vi "Front Panel.vi"(11 "GUI In":refnum<class "Humidity Profile UI.lvclass">) -> ()   [LabVIEW 2015, in "Humidity Profile UI.lvclass"]
uses:
  Humidity Profile UI.lvclass
  Seq.ctl
  Humidity Profile/Change Temperature/Change Temperature.lvclass
  Reusable/GUI/GUI.lvclass/GUI.ctl
  Reusable/Observer/Observer.lvclass/Observer.ctl
  Reusable/Sequence/SEQ/SEQ.lvclass
  Reusable/Sequence/STEPS/STEP.lvclass
  Humidity Profile/Change PAS Flow/Change PAS Flow.lvclass
  Reusable/Sequence/STEPS/LEAVES/Double/Switch DBL.lvclass/Switch DBL.ctl
  Humidity Profile/Change QmRH/Change QmRH.lvclass
  Calibration/Change Filter State/Change Filter Position.lvclass
  Humidity Profile/Change Flow/Change Flow.lvclass
  Calibration/Wait/Wait.lvclass
  Calibration/Wait/Wait.lvclass/Wait.ctl
  Controls/MFC Address.ctl
  CRDS/Data/cCRDS Data.lvclass
  Reusable/Sequence/STEPS/LEAVES/Double/Write val.vi
  Calibration/Wait/Write Wait Time.vi
  Reusable/GUI/Accessors/Read RegEvent.vi
  Reusable/Observer/Read Data Queue.vi
  CRDS/Data/Read vData.vi
  CRDS/Data/Read Humidifier T.vi
  Reusable/Data/Data.lvclass
panel:
  in  "cSequence":bool
  in  "lSequence":bool
  in  "saveSeq":bool
  out "Alicat Data":T1
  out "T":sgl
  in  "run":bool
  in  "T":sgl caption="T (degC)"
  in  "Q":sgl caption="Qclap (lpm)"
  out "seqMsg":string[](array[string]) caption="Messages"
  in  "Steps":string[](tree)
  in  "Sequence":string(tree)
  # "This user interface is used to handle the profiling of humidities.  The system handles three different humidified channels.  The temperature handled on this page is the temperature associated with the medium RH channel.  The flow controls the dilution flow to the mixing tank between the high humidity channel and the channel that the thermal denuded channel.  This flow is directly connected to the high humidity flow control on the CRD page."
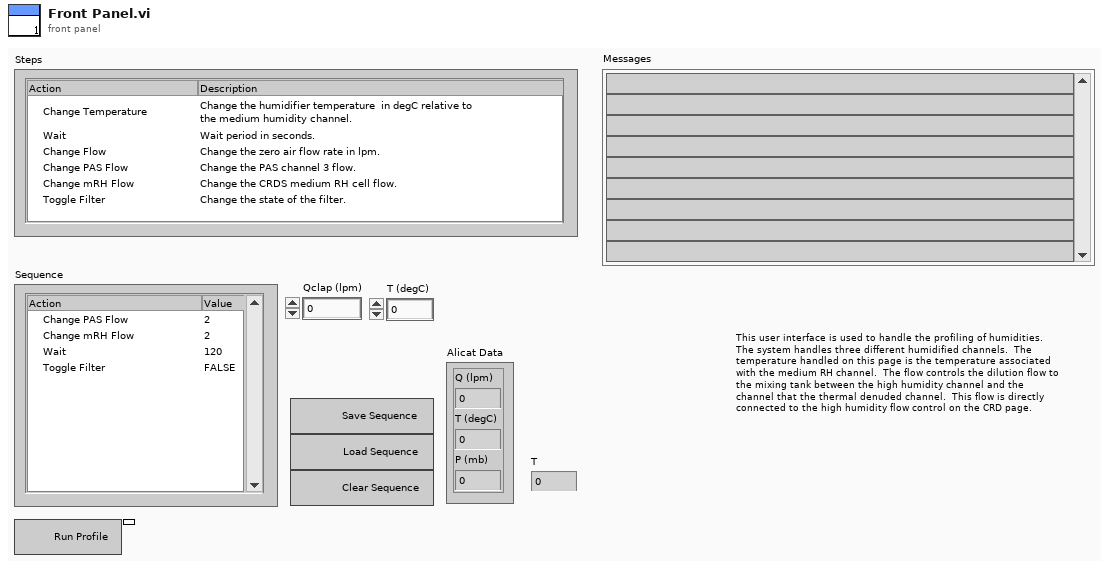
[diagram p1: front panel]
types:
  T1 = cluster{"Q (lpm)":dbl, "T (degC)":dbl, "P (mb)":dbl}
  T2 = typedef "Seq.ctl" = enum16{"Load Sequence", "Run Sequence", "Stop Sequence", "Do Nothing"}
  T3 = cluster{"Numeric":sgl, "Numeric":sgl, "Numeric":sgl}
  T4 = typedef "eventvkey.ctl" = enum16{"ASCII", "Enter", "Return", "Shift", "Ctrl", "Alt", "Cmd", "Opt", "Caps", "NumLock", "Clear", "Break", "Up", "Down", "Left", "Right", "Insert", "Delete", "Home", "End", "PageUp", "PageDown", "Escape", "Help", "Pause", "ScrollLock", "F1", "F2", "F3", "F4", "F5", "F6", "F7", "F8", "F9", "F10", "F11", "F12", "F13", "F14", "F15", "F16", "F17", "F18", "F19", "F20", "F21", "F22", "F23", "F24", "Play", "VolumeUp", "VolumeDown", "Mute", "Two Byte Char"}
  T5 = enum16{"Load Sequence", "Run Sequence", "Stop Sequence"}
  T6 = typedef "MFC Address.ctl" = enum16{"CRDS Purge", "CRDS Thermodenuded", "CRDS Dry", "CRDS Med RH", "CRDS High RH", "PAS Ch 1", "PAS Ch 2", "PAS Ch3", "PAS Ch 4", "PAS Ch 5", "CLAP", "O3", "Pinlet"}
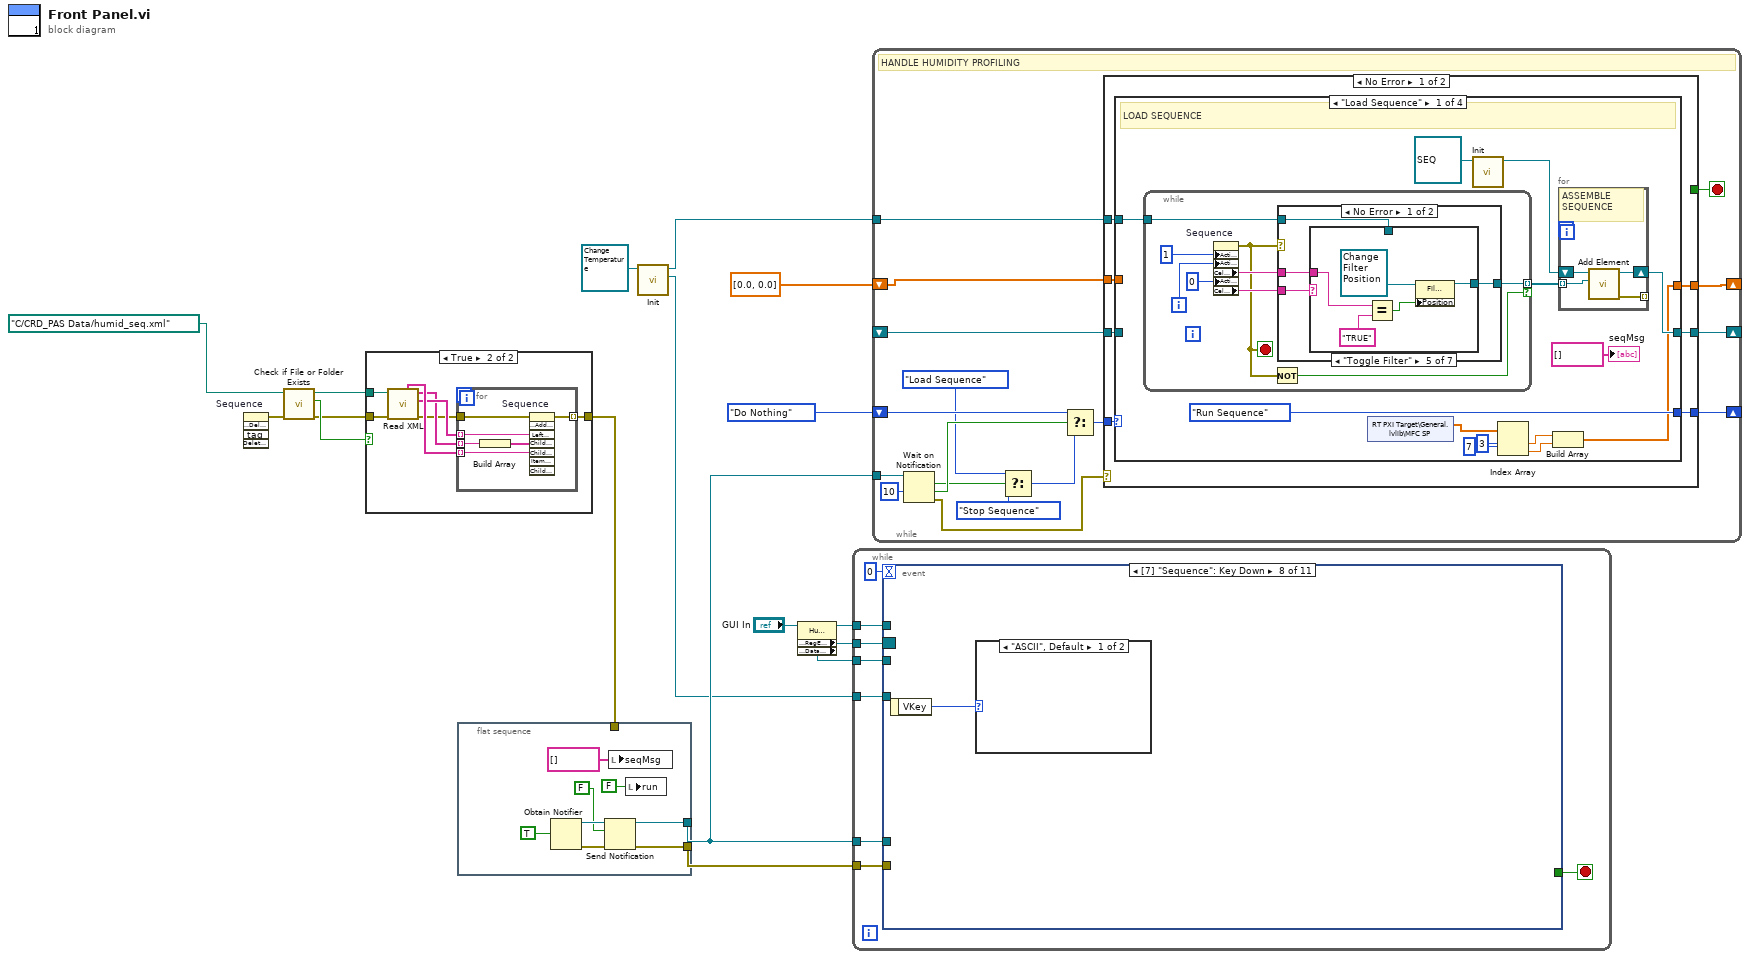
[diagram p0: block diagram]
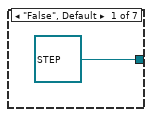
[diagram p3: hidden frame]
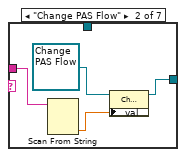
[diagram p4: hidden frame]
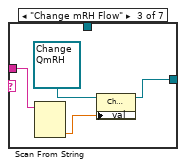
[diagram p5: hidden frame]
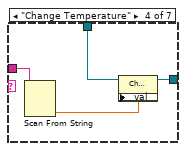
[diagram p6: hidden frame]
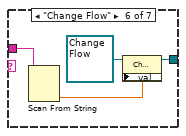
[diagram p7: hidden frame]
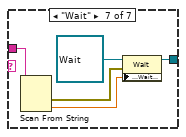
[diagram p8: hidden frame]
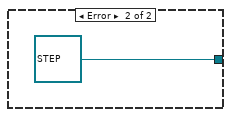
[diagram p9: hidden frame]
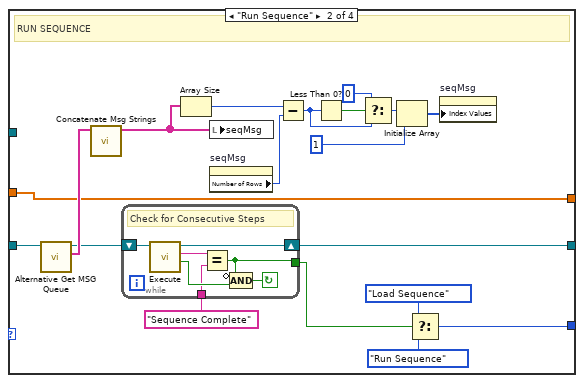
[diagram p10: hidden frame]
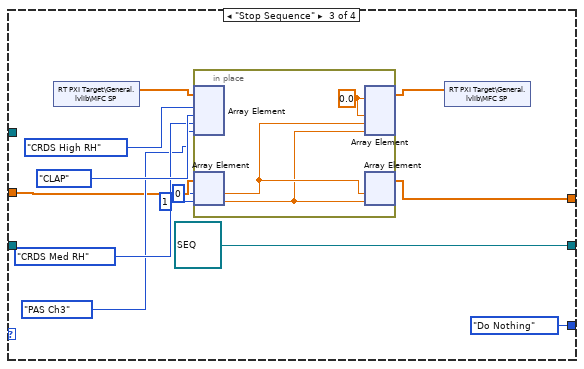
[diagram p11: hidden frame]
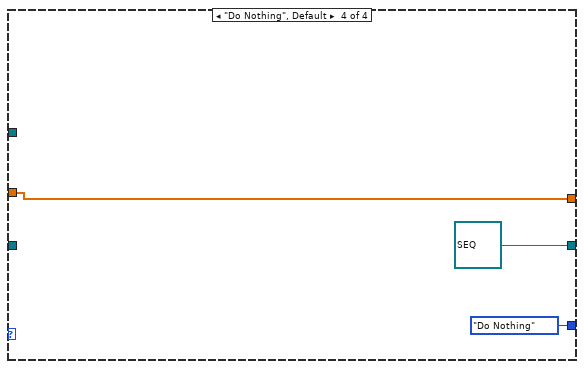
[diagram p12: hidden frame]
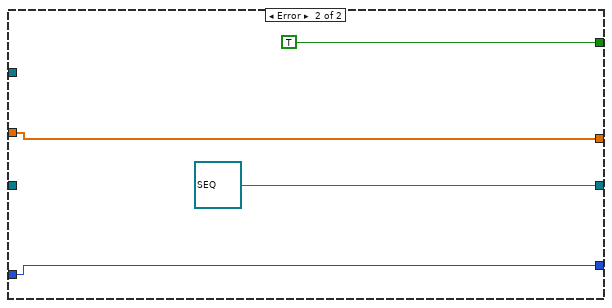
[diagram p13: hidden frame]
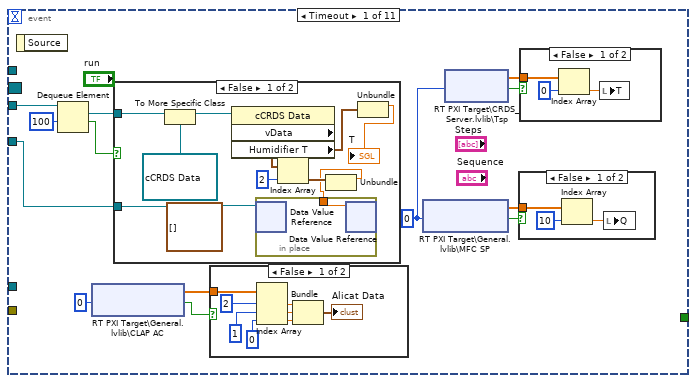
[diagram p14: hidden frame]
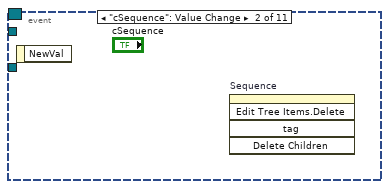
[diagram p19: hidden frame]
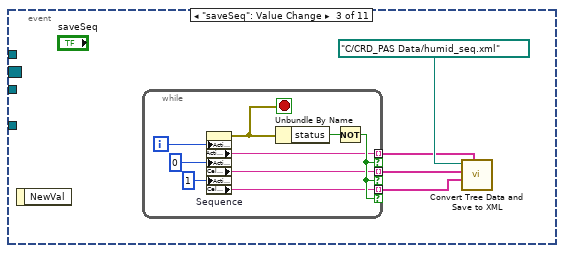
[diagram p20: hidden frame]
diagram:
  n1 = invoke on="Sequence" class="Tree (strict)" method="Edit Tree Items.Delete"() -> (error out=w9:errorcluster)  [unwired: 5 in, 4 out]
  n2 = call <vilib>:"Check if File or Folder Exists.vi"("error in (no error)"=w9, "path"=path "C:/CRD_PAS Data/humid_seq.xml" ("file")) -> ("error out"=w8:errorcluster, "file or folder exists?"=w10:bool, "dup path"=w7:path)  [unwired: 7 in]
  n3 = case shown="True" w10 {
    tunnel: w8 -> [_ w20]
    tunnel: w7 -> [_ w22]
    tunnel: [_ w18] -> w5
    frame False {
    }
    frame True {
      n4 = call "Read XML.vi"("error in"=w20, "path"=w22) -> ("error out"=w19:errorcluster, "Steps"=w23:string[], "Values"=w21:string[], "tags"=w24:string[])  [unwired: 5 in, 1 out]
      n5 = for {
        tunnel: w24 -> [w30] mode=indexing
        tunnel: w23 -> [w29] mode=indexing
        tunnel: w21 -> [w28] mode=indexing
        tunnel: w19 -> [w26]
        tunnel: [w25] -> w18 mode=indexing
        n6 = Build Array(w28) -> (w27:string[])
        n7 = invoke on="Sequence" class="Tree (strict)" method="Edit Tree Items.Add Item to End"(error in=w26, "Left Cell"=w29, "Child Text"=w27, "Child Tag"=w30) -> (error out=w25:errorcluster)  [unwired: 4 in, 7 out]
      }
    }
  }
  n8 = flat-sequence {
    tunnel: [w34] -> w14
    tunnel: [w33] -> w13
    tunnel: w5 -> [_]
    frame #0 {
      n9 = Obtain Notifier(notification data type=TRUE) -> (notifier out=w37:refnum<notifier>, error out=w36:errorcluster)  [unwired: 3 in, 1 out]
      n10 = Send Notification(notification=FALSE, notifier=w37, error in (no error)=w36) -> (notifier out=w33:refnum<notifier>, error out=w34:errorcluster)
      n11 = local write "seqMsg"(string[] [] ("seqMsg")) -> ()
      n12 = local write "run"(FALSE ("run")) -> ()
    }
  }
  n13 = call "Init.vi"("Change Temperature in"=refnum<class "Change Temperature.lvclass"> refnum) -> ("T DVR"=w2:refnum<data-value>, "Change Temperature out"=w3:refnum<class "Change Temperature.lvclass">)  [unwired: 8 in, 1 out]
  n14 = property class="Humidity Profile"(reference="GUI In") -> (reference out=w11:refnum<class "Humidity Profile UI.lvclass">, "Data Access:RegEvent"=w16:refnum<event-registration>, "Data Access:Data Queue"=w15:refnum<queue>)  [unwired: 1 in, 1 out]
  n15 = while {
    tunnel: w16 -> [w46]
    tunnel: w15 -> [w44]
    tunnel: w13 -> [w43]
    tunnel: w14 -> [w42]
    tunnel: w11 -> [w40]
    tunnel: w2 -> [w39]
    stop <- w45 stop-if-true
    n16 = event shown="[7] \"Sequence\": Key Down" {
      selector: w46 -> [_ _ _ _ _ _ _ _ _ _ _]
      dyn-events: _ -> [_ _ _ _ _ _ _ _ _ _ _]
      timeout: 0 -> [_ _ _ _ _ _ _ _ _ _ _]
      tunnel: [_ _ _ _ _ _ _ _ TRUE _ _] -> w45
      tunnel: w44 -> [w59 _ _ _ _ _ _ _ _ _ _]
      tunnel: w43 -> [_ _ _ _ w119 _ _ _ w136 _ _]
      tunnel: w42 -> [_ _ _ _ w118 _ _ _ w135 _ _]
      tunnel: w40 -> [_ _ _ _ _ _ _ _ w134 _ _]
      tunnel: w39 -> [w47 _ _ _ _ _ _ _ w133 _ _]
      event Timeout {
        w52 = 0 ("ms timeout (0)")
        n17 = event-data() -> ()  [unwired: 1 in, 1 out]
        n18 = Dequeue Element(queue=w59, timeout in ms (-1)=100) -> (element=w58:refnum<data-value>, timed out?=w53:bool)  [unwired: 1 in, 2 out]
        n19 = shared-variable "RT PXI Target\\General.lvlib\\CLAP AC"(0 ("ms timeout (0)")) -> (w51:sgl[], w49:bool)  [unwired: 1 in, 1 out]
        n20 = case shown="False" w53 {
          tunnel: w58 -> [w77 _]
          tunnel: w47 -> [w74 _]
          frame False {
            (unwired) cluster{"TRH":dbl, "RH":dbl}[] [] ("vData")
            n21 = To More Specific Class(target class=refnum<data-value> refnum ("element"), reference=w77) -> (specific class reference=w75:refnum<data-value>)  [unwired: 1 in, 1 out]
            n22 = property class="cCRDS Data"(reference=w75) -> ("vData"=w73:cluster{"TRH":dbl, "RH":dbl}[], "Humidifier T"=w69:cluster{"Hum 1":sgl, "Hum 2":sgl})  [unwired: 1 in, 2 out]
            n23 = Index Array(array=w73, index=2) -> (element=w71:cluster{"TRH":dbl, "RH":dbl})
            n24 = Unbundle(w71) -> ("TRH"=w70:dbl)  [unwired: 1 out]
            n25 = in-place {
              in-place-border: w70 -> [w78]
              n26 = in-place-dvr #1(w74) -> ()  [unwired: 2 out]
              n27 = in-place-dvr #1(w78) -> ()  [unwired: 2 out]
            }
            n28 = Unbundle(w69) -> ("Hum 1"=→"T":sgl)  [unwired: 1 out]
          }
          frame True {
          }
        }
        n29 = case shown="False" w49 {
          tunnel: w51 -> [w61 _]
          frame False {
            n30 = Index Array(array=w61, index #1=2 ("index"), index #2=1 ("index"), index #3=0 ("index")) -> (element #1=w65:sgl, element #2=w66:sgl, element #3=w67:sgl)
            n31 = Bundle("Numeric"=w65, "Numeric"=w66, "Numeric"=w67) -> (→"Alicat Data":T3)  [unwired: 1 in]
          }
          frame True {
          }
        }
        n32 = shared-variable "RT PXI Target\\General.lvlib\\MFC SP"(w52) -> (w54:sgl[], w55:bool)  [unwired: 1 in, 1 out]
        n33 = shared-variable "RT PXI Target\\CRDS_Server.lvlib\\Tsp"(w52) -> (w56:sgl[], w57:bool)  [unwired: 1 in, 1 out]
        n34 = case shown="False" w55 {
          tunnel: w54 -> [w81 _]
          frame False {
            n35 = Index Array(array=w81, index=10) -> (element=w79:sgl)
            n36 = local write "Q"(w79) -> ()
          }
          frame True {
          }
        }
        n37 = case shown="False" w57 {
          tunnel: w56 -> [w84 _]
          frame False {
            n38 = Index Array(array=w84, index=0) -> (element=w82:sgl)
            n39 = local write "T"(w82) -> ()
          }
          frame True {
          }
        }
      }
      event "cSequence": Value Change {
        n40 = event-data() -> ()  [unwired: 1 in, 1 out]
        n41 = invoke on="Sequence" class="Tree (strict)" method="Edit Tree Items.Delete"() -> ()  [unwired: 5 in, 5 out]
      }
      event "saveSeq": Value Change {
        n42 = event-data() -> ()  [unwired: 1 in, 1 out]
        n43 = while {
          tunnel: [w93] -> w87 mode=indexing if=w94
          tunnel: [w90] -> w86 mode=indexing if=w94
          tunnel: [w89] -> w85 mode=indexing if=w94
          i -> [w92]
          stop <- w96 stop-if-true
          n44 = property on="Sequence" class="Tree (strict)"("Active Item Row Number"=w92, "ActiveColNum"=0 ("Active Cell:Active Column Number"), "ActiveColNum"=1 ("Active Cell:Active Column Number")) -> (error out=w96:errorcluster, "Active Item Tag"=w93:string, "Cell String"=w90:string, "Cell String"=w89:string)  [unwired: 2 in, 1 out]
          n45 = Unbundle By Name(w96) -> ("status"=w97:bool)
          n46 = Not(x=w97) -> (.not. x?=w94:bool)
        }
        n47 = call "Convert Tree Data and Save to XML.vi"("tag"=w87, "Value"=w85, "Step"=w86, "file"=path "C:/CRD_PAS Data/humid_seq.xml") -> ()  [unwired: 5 in, 3 out]
      }
      event "lSequence": Value Change {
        n48 = event-data() -> ()  [unwired: 1 in, 1 out]
        n49 = call "File Dialog"("prompt"="Open sequence file.", "pattern (all files)"="*.xml") -> ("selected path"=w101:path, "cancelled"=w99:bool, "error out"=w98:errorcluster)  [unwired: 10 in, 1 out]
        n50 = case shown="False" w99 {
          tunnel: w101 -> [w108 _]
          tunnel: [w105 _] -> _
          tunnel: w98 -> [w104 _]
          frame False {
            n51 = invoke on="Sequence" class="Tree (strict)" method="Edit Tree Items.Delete"(error in=w104) -> (error out=w103:errorcluster)  [unwired: 4 in, 4 out]
            n52 = call "Read XML.vi"("error in"=w103, "path"=w108) -> ("error out"=w106:errorcluster, "Steps"=w109:string[], "Values"=w107:string[], "tags"=w110:string[])  [unwired: 5 in, 1 out]
            n53 = for {
              tunnel: w110 -> [w116] mode=indexing
              tunnel: w109 -> [w115] mode=indexing
              tunnel: w107 -> [w114] mode=indexing
              tunnel: w106 -> [w112]
              tunnel: [w111] -> w105 mode=indexing
              n54 = Build Array(w114) -> (w113:string[])
              n55 = invoke on="Sequence" class="Tree (strict)" method="Edit Tree Items.Add Item to End"(error in=w112, "Left Cell"=w115, "Child Text"=w113, "Child Tag"=w116) -> (error out=w111:errorcluster)  [unwired: 4 in, 7 out]
            }
          }
          frame True {
          }
        }
      }
      event "run": Value Change {
        n56 = event-data() -> ("NewVal"=w117:bool)  [unwired: 1 in]
        n57 = Send Notification(notification=w117, notifier=w119, error in (no error)=w118) -> ()  [unwired: 2 out]
      }
      event "Q": Value Change {
        n58 = event-data() -> ()  [unwired: 1 in, 1 out]
        n59 = shared-variable "RT PXI Target\\General.lvlib\\MFC SP"() -> (w122:sgl[])  [unwired: 1 in, 1 out]
        n60 = in-place {
          in-place-border: "Q" -> [w124]
          n61 = in-place-array #2(w122, 10) -> ()  [unwired: 1 out]
          n62 = in-place-array #2(w124) -> (w120:sgl[])  [unwired: 1 out]
        }
        n63 = shared-variable "RT PXI Target\\General.lvlib\\MFC SP"(w120) -> ()  [unwired: 1 in, 1 out]
      }
      event "T": Value Change {
        n64 = event-data() -> ()  [unwired: 1 in, 1 out]
        n65 = shared-variable "RT PXI Target\\CRDS_Server.lvlib\\Tsp"() -> (w128:sgl[])  [unwired: 1 in, 1 out]
        n66 = in-place {
          in-place-border: "T" -> [w129]
          n67 = in-place-array #3(w128, 0) -> ()  [unwired: 1 out]
          n68 = in-place-array #3(w129) -> (w125:sgl[])  [unwired: 1 out]
        }
        n69 = shared-variable "RT PXI Target\\CRDS_Server.lvlib\\Tsp"(w125) -> ()  [unwired: 1 in, 1 out]
      }
      event "Sequence": Key Down {
        n70 = event-data() -> ("VKey"=w130:T4)  [unwired: 1 in]
        n71 = case shown="\"ASCII\", Default" w130 {
          frame "ASCII", Default {
          }
          frame "Delete" {
            n72 = local read "Sequence"() -> (w132:string)
            n73 = invoke on="Sequence" class="Tree (strict)" method="Edit Tree Items.Delete"("tag"=w132, "Delete Children"=TRUE ("Delete Children?")) -> ()  [unwired: 3 in, 5 out]
          }
        }
      }
      event User Event; Panel Close {
        n74 = event-data() -> ()  [unwired: 1 in, 1 out]
        n75 = call-dynamic "Stop FP.vi"("GUI in"=w134) -> ()  [unwired: 9 in, 2 out]
        n76 = Release Notifier(notifier=w136, error in (no error)=w135) -> ()  [unwired: 1 in, 3 out]
        n77 = Delete Data Value Reference(data value reference=w133) -> ()  [unwired: 1 in, 2 out]
      }
      event "Steps": Double Click {
        n78 = event-data() -> ("Tag"=w141:string)  [unwired: 1 in]
        n79 = property on="Steps" class="Tree (strict)"("Active Item Tag"=w141, "ActiveColNum"=0 ("Active Cell:Active Column Number")) -> ("Cell String"=w143:string, "Active Item Tag"=w140:string)  [unwired: 2 in, 2 out]
        n80 = case shown="\"filter\"" w140 {
          tunnel: ["0" "FALSE"] -> w139
          frame "False", Default {
          }
          frame "filter" {
          }
        }
        n81 = Build Array(w139) -> (w138:string[])
        n82 = invoke on="Sequence" class="Tree (strict)" method="Edit Tree Items.Add Item to End"("Left Cell"=w143, "Child Text"=w138, "Child Tag"=w140, "Item Indent"=0 ("New Item Indentation")) -> ()  [unwired: 4 in, 8 out]
      }
      event "Steps": Key Down {
        n83 = event-data() -> ("VKey"=w147:T4)  [unwired: 1 in]
        n84 = case shown="\"Enter\"" w147 {
          frame "ASCII", Default {
          }
          frame "Enter" {
            n85 = property on="Steps" class="Tree (strict)"() -> ("Active Item Tag"=w148:string)  [unwired: 2 in, 2 out]
            n86 = property on="Steps" class="Tree (strict)"("Active Item Tag"=w148, "ActiveColNum"=0 ("Active Cell:Active Column Number")) -> ("Cell String"=w151:string, "Active Item Tag"=w153:string)  [unwired: 2 in, 2 out]
            n87 = invoke on="Sequence" class="Tree (strict)" method="Edit Tree Items.Add Item to End"("Left Cell"=w151, "Child Text"=string[] ["0"], "Child Tag"=w153, "Item Indent"=0 ("New Item Indentation")) -> ()  [unwired: 4 in, 8 out]
          }
        }
      }
    }
  }
  n88 = while {
    shift-right: [w170] -> _
    shift-left: _ -> [w169]
    tunnel: w13 -> [w168]
    shift-right: [w165] -> _
    shift-left: Seq."Do Nothing" -> [w160]
    tunnel: w3 -> [w156]
    shift-right: [w154] -> _
    shift-left: sgl[] [0.0, 0.0] -> [w155]
    stop <- w166 stop-if-true
    # "HANDLE HUMIDITY PROFILING"
    n89 = Wait on Notification(notifier=w168, timeout in ms (-1)=10) -> (notification=w162:bool, timed out?=w163:bool, error out=w167:errorcluster)  [unwired: 2 in, 1 out]
    n90 = Select(t=Seq."Load Sequence", s=w162, f=Seq."Stop Sequence") -> (s? t:f=w161:T2)
    n91 = Select(t=w160, s=w163, f=w161) -> (s? t:f=w159:T2)
    n92 = case shown="No Error" w167 {
      tunnel: [w177 refnum<class "SEQ.lvclass"> refnum ("SEQ out")] -> w170
      tunnel: w169 -> [w176 _]
      tunnel: [_ TRUE] -> w166
      tunnel: [w175 w281] -> w165
      tunnel: w159 -> [w174 w281]
      tunnel: w156 -> [w173 _]
      tunnel: w155 -> [w172 w280]
      tunnel: [w171 w280] -> w154
      frame No Error {
        n93 = case shown="\"Load Sequence\"" w174 {
          tunnel: [w187 w245 refnum<class "SEQ.lvclass"> refnum ("New Sequence") refnum<class "SEQ.lvclass"> refnum ("New Sequence")] -> w177
          tunnel: w176 -> [_ w244 _ _]
          tunnel: [Seq."Run Sequence" w238 Seq."Do Nothing" Seq."Do Nothing"] -> w175
          tunnel: w173 -> [w184 _ _ _]
          tunnel: w172 -> [_ w236 w265 w277]
          tunnel: [w178 w236 w262 w277] -> w171
          frame "Load Sequence" {
            # "LOAD SEQUENCE"
            n94 = while {
              tunnel: [w198] -> w188 mode=indexing if=w196
              tunnel: w184 -> [w195]
              i -> [w202]
              stop <- w197 stop-if-true
              n95 = property on="Sequence" class="Tree (strict)"("ActiveColNum"=1 ("Active Cell:Active Column Number"), "Active Item Row Number"=w202, "ActiveColNum"=0 ("Active Cell:Active Column Number")) -> (error out=w197:errorcluster, "Cell String"=w199:string, "Cell String"=w200:string)  [unwired: 2 in, 1 out]
              n96 = Not(x=w197) -> (.not. x?=w196:bool)
              n97 = case shown="No Error" w197 {
                tunnel: w200 -> [w207 _]
                tunnel: w199 -> [w206 _]
                tunnel: [w205 refnum<class "STEP.lvclass"> refnum ("Sequence Composition:STEP.lvclass")] -> w198
                tunnel: w195 -> [w204 _]
                frame No Error {
                  n98 = case shown="\"Toggle Filter\"" w207 {
                    tunnel: [refnum<class "STEP.lvclass"> refnum ("Sequence Composition:STEP.lvclass") w209 w213 w219 w224 w226 w232] -> w205
                    tunnel: w206 -> [_ w211 w215 w220 w223 w228 w230]
                    tunnel: w204 -> [_ _ _ w217 _ _ _]
                    frame "False", Default {
                    }
                    frame "Change PAS Flow" {
                      n99 = Scan From String(input string=w211) -> (output 1=w212:dbl)  [unwired: 4 in, 3 out]
                      n100 = property class="Change PAS Flow.lvclass"(reference=refnum<class "Change PAS Flow.lvclass"> refnum ("Change PAS Flow.lvclass"), "val"=w212) -> (reference out=w209:refnum<class "Change PAS Flow.lvclass">)  [unwired: 1 in, 1 out]
                    }
                    frame "Change mRH Flow" {
                      n101 = Scan From String(input string=w215) -> (output 1=w214:dbl)  [unwired: 4 in, 3 out]
                      n102 = property class="Change QmRH.lvclass"(reference=refnum<class "Change QmRH.lvclass"> refnum ("Change QmRH.lvclass"), "val"=w214) -> (reference out=w213:refnum<class "Change QmRH.lvclass">)  [unwired: 1 in, 1 out]
                    }
                    frame "Change Temperature" {
                      n103 = Scan From String(input string=w220) -> (output 1=w218:dbl)  [unwired: 4 in, 3 out]
                      n104 = property class="Change Temperature"(reference=w217, "val"=w218) -> (reference out=w219:refnum<class "Change Temperature.lvclass">)  [unwired: 1 in, 1 out]
                    }
                    frame "Toggle Filter" {
                      n105 = Equal?(x=w223, y="TRUE") -> (x = y?=w221:bool)
                      n106 = property class="Filter Position"(reference=refnum<class "Change Filter Position.lvclass"> refnum ("Filter Position"), "Position"=w221) -> (reference out=w224:refnum<class "Change Filter Position.lvclass">)  [unwired: 1 in, 1 out]
                    }
                    frame "Change Flow" {
                      n107 = Scan From String(input string=w228) -> (output 1=w227:dbl)  [unwired: 4 in, 3 out]
                      n108 = property class="Change Flow"(reference=refnum<class "Change Flow.lvclass"> refnum ("Change Flow"), "val"=w227) -> (reference out=w226:refnum<class "Change Flow.lvclass">)  [unwired: 1 in, 1 out]
                    }
                    frame "Wait" {
                      n109 = Scan From String(input string=w230) -> (error out=w231:errorcluster, output 1=w233:dbl)  [unwired: 4 in, 2 out]
                      n110 = property class="Wait"(reference=refnum<class "Wait.lvclass"> refnum ("Wait"), error in=w231, "Data Access:Wait Time"=w233) -> (reference out=w232:refnum<class "Wait.lvclass">)  [unwired: 1 out]
                    }
                  }
                }
                frame Error {
                }
              }
            }
            n111 = shared-variable "RT PXI Target\\General.lvlib\\MFC SP"() -> (w183:sgl[])  [unwired: 1 in, 1 out]
            n112 = call-dynamic "Init.vi"("SEQ in"=refnum<class "SEQ.lvclass"> refnum) -> ("SEQ out"=w189:refnum<class "SEQ.lvclass">)  [unwired: 9 in, 1 out]
            n113 = Index Array(array=w183, index #1=3 ("index"), index #2=7 ("index")) -> (element #1=w180:sgl, element #2=w179:sgl)
            n114 = Build Array(w180, w179) -> (w178:sgl[])
            n115 = for {
              shift-right: [w194] -> w187
              shift-left: w189 -> [w192]
              tunnel: [w193] -> _ mode=indexing
              tunnel: w188 -> [w191] mode=indexing
              # "ASSEMBLE SEQUENCE"
              n116 = call "Add Element.vi"("STEP"=w191, "SEQ in"=w192) -> ("error out"=w193:errorcluster, "SEQ out"=w194:refnum<class "SEQ.lvclass">)  [unwired: 8 in]
            }
            "seqMsg" <- string[] [] ("seqMsg")
          }
          frame "Run Sequence" {
            # "RUN SEQUENCE"
            n117 = call "Alternative Get MSG Queue.vi"("SEQ in"=w244) -> ("seqMsg"=w247:string[], "SEQ Out"=w237:refnum<class "SEQ.lvclass">)  [unwired: 8 in, 1 out]
            n118 = call "Concatenate Msg Strings.vi"("StringsIn"=w247) -> ("StringsOut"=w248:string[])  [unwired: 10 in]
            n119 = while {
              shift-right: [w260] -> w245
              shift-left: w237 -> [w261]
              tunnel: "Sequence Complete" ("t") -> [w257]
              tunnel: [w255] -> w241
              stop <- w256 continue-if-true
              # "Check for Consecutive Steps"
              n120 = call-dynamic "Execute.vi"("SEQ in"=w261) -> ("Next Step?"=w258:bool, "MSG"=w259:string, "SEQ out"=w260:refnum<class "SEQ.lvclass">)  [unwired: 7 in, 1 out]
              n121 = Equal?(x=w259, y=w257) -> (x = y?=w255:bool)
              n122 = Compound Arithmetic op=AND(invert w255, w258) -> (w256:bool)
            }
            n123 = Array Size(array=w248) -> (size(s)=w254:i32)
            n124 = local write "seqMsg"(w248) -> ()
            n125 = property on="seqMsg" class="Arr (strict)"() -> ("Number of Rows"=w243:u32)  [unwired: 2 in, 2 out]
            n126 = Subtract(x=w254, y=w243) -> (x-y=w251:u32)
            n127 = Less Than 0?(x=w251) -> (x < 0?=w252:bool)
            n128 = Select(t=u32 0, s=w252, f=w251) -> (s? t:f=w249:u32)
            n129 = Initialize Array(w249, 1 ("dimension size")) -> (w242:u32[])
            n130 = Select(t=T5."Load Sequence", s=w241, f=T5."Run Sequence") -> (s? t:f=w238:T5)
            n131 = property on="seqMsg" class="Arr (strict)"("Index Values"=w242) -> ()  [unwired: 2 in, 2 out]
          }
          frame "Stop Sequence" {
            n132 = shared-variable "RT PXI Target\\General.lvlib\\MFC SP"() -> (w272:sgl[])  [unwired: 1 in, 1 out]
            n133 = in-place {
              w276 = sgl 0.0 ("element")
              n134 = in-place-array #4(w272, MFC_Address."CRDS High RH" ("Controllers"), MFC_Address."CLAP" ("Controllers"), MFC_Address."CRDS Med RH" ("Controllers"), MFC_Address."PAS Ch3" ("Controllers")) -> ()  [unwired: 4 out]
              n135 = in-place-array #5(w265, 0, 1) -> (w275:sgl, w274:sgl)
              n136 = in-place-array #4(w276, w276, w275, w274) -> (w269:sgl[])  [unwired: 4 out]
              n137 = in-place-array #5(w275, w274) -> (w262:sgl[])  [unwired: 2 out]
            }
            n138 = shared-variable "RT PXI Target\\General.lvlib\\MFC SP"(w269) -> ()  [unwired: 1 in, 1 out]
          }
          frame "Do Nothing", Default {
          }
        }
      }
      frame Error {
      }
    }
  }
